vi "Write base.vi"(8 "error in (no error)":errorcluster, 10 "base":dbl, 11 "Solution Triangle in":refnum<class "Solution Triangle.lvclass">) -> (0 "error out":errorcluster, 3 "Solution Triangle out":refnum<class "Solution Triangle.lvclass">)   [LabVIEW 2015, in "Solution Triangle.lvclass"]
uses:
  Solution Triangle.lvclass
  Solution Triangle.lvclass/Solution Triangle.ctl
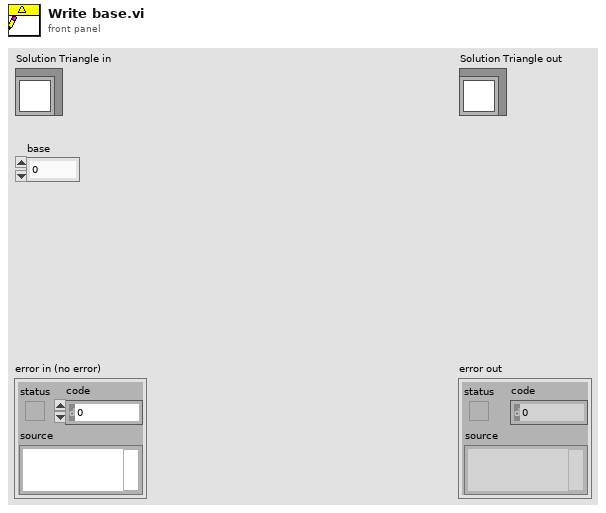
[diagram p1: front panel]
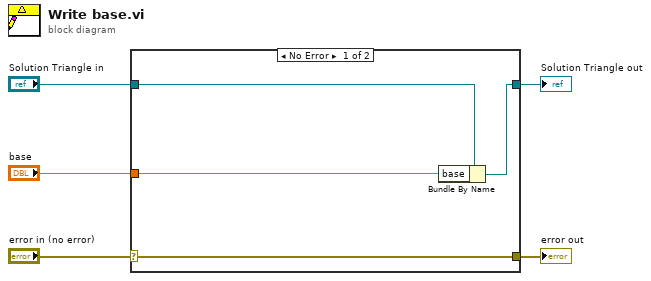
[diagram p0: block diagram]
diagram:
  n1 = case shown="No Error" "error in (no error)" {
    selector: "error in (no error)" -> [w9 w10]
    tunnel: [w9 w10] -> w4
    tunnel: [w7 w11] -> w2
    tunnel: "Solution Triangle in" -> [w8 w11]
    tunnel: "base" -> [w6 _]
    frame No Error {
      n2 = Bundle By Name(cluster=w8, "base"=w6) -> (w7:refnum<class "Solution Triangle.lvclass">)
    }
    frame Error {
    }
  }
  "error out" <- w4
  "Solution Triangle out" <- w2
